vi "Set connection string.vi"(8 "error in (no error)":errorcluster, 11 "database in":refnum<class "database.lvclass">) -> (0 "error out":errorcluster, 3 "database out":refnum<class "database.lvclass">)   [LabVIEW 2018, in "database.lvclass"]
uses:
  database.lvclass
  database.lvclass/database.ctl
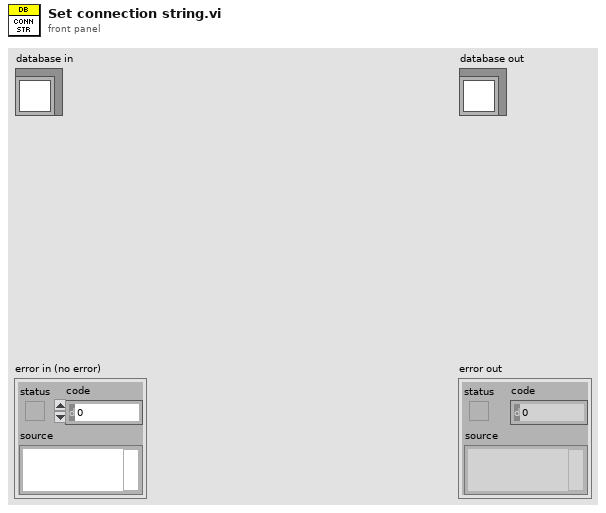
[diagram p1: front panel]
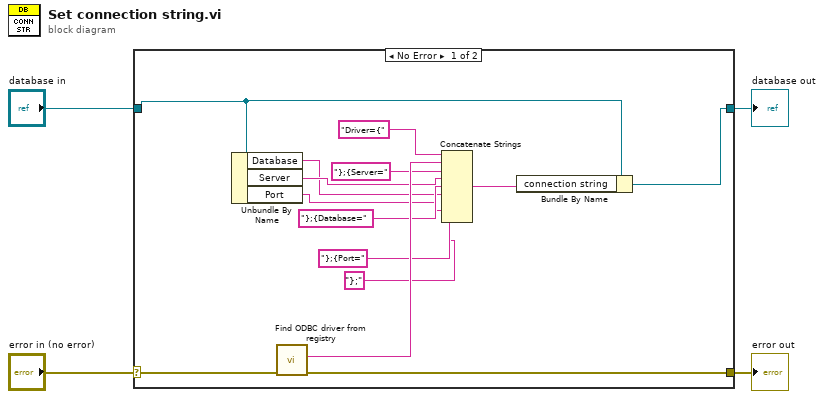
[diagram p0: block diagram]
diagram:
  n1 = case shown="No Error" "error in (no error)" {
    selector: "error in (no error)" -> [w16 w20]
    tunnel: [w15 w20] -> w3
    tunnel: [w18 w19] -> w1
    tunnel: "database in" -> [w17 w19]
    frame No Error {
      n2 = Unbundle By Name(w17) -> ("Database"=w9:string, "Server"=w11:string, "Port"=w7:string)
      n3 = call "Find ODBC driver from registry.vi"("error in (no error)"=w16) -> ("error out"=w15:errorcluster, "driver"=w13:string)  [unwired: 9 in]
      n4 = Concatenate Strings("Driver={" ("string"), w13, "};{Server=" ("string"), w11, "};{Database=" ("string"), w9, "};{Port=" ("string"), w7, "};" ("string")) -> (w5:string)
      n5 = Bundle By Name(cluster=w17, "connection string"=w5) -> (w18:refnum<class "database.lvclass">)
    }
    frame Error {
    }
  }
  "error out" <- w3
  "database out" <- w1
